vi "Sweeping Turn.vi"(6 "upper angle limit":dbl, 8 "error in":errorcluster) -> (0 "error out":errorcluster)   [LabVIEW 2017]
uses:
  Documents/LabVIEW Data/Retro 2018/Robot Global Data.vi
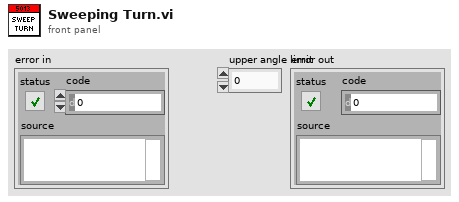
[diagram p1: front panel]
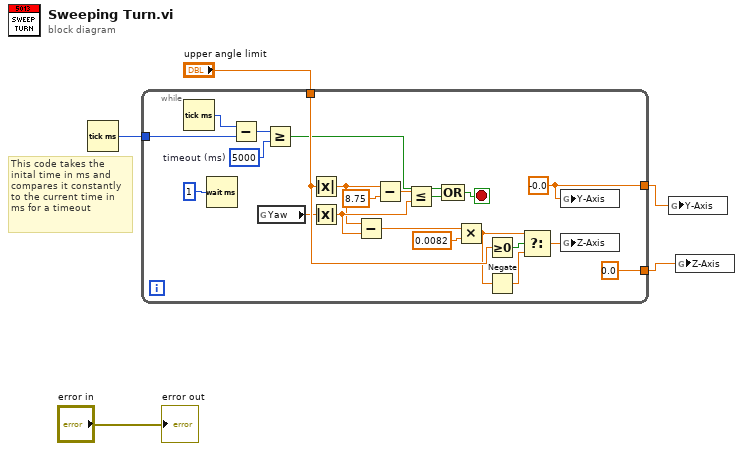
[diagram p0: block diagram]
diagram:
  # "This code takes the\ninital time in ms and\ncompares it constantly\nto the current time in\nms for a timeout"
  n1 = Tick Count (ms)() -> (millisecond timer value=w1:u32)
  n2 = while {
    tunnel: "upper angle limit" -> [w24]
    tunnel: [0.0 ("setpoint")] -> w3
    tunnel: [w17] -> w2
    tunnel: w1 -> [w10]
    stop <- w8 stop-if-true
    w6 = u32 5000  # timeout (ms)
    w17 = -0.0 ("Y-Axis")
    n3 = Tick Count (ms)() -> (millisecond timer value=w11:u32)
    n4 = Wait (ms)(milliseconds to wait=u32 1) -> ()  [unwired: 1 out]
    n5 = Subtract(x=w11, y=w10) -> (x-y=w9:u32)
    n6 = global read "Robot Global Data.vi" "Yaw"() -> (w18:dbl)
    n7 = Greater Or Equal?(x=w9, y=w6) -> (x >= y?=w7:bool)
    n8 = Absolute Value(x=w24) -> (abs(x)=w15:dbl)
    n9 = Absolute Value(x=w18) -> (abs(x)=w16:dbl)
    n10 = Subtract(x=w15, y=w16) -> (x-y=w14:dbl)
    n11 = Subtract(x=w15, y=8.75 ("x")) -> (x-y=w20:dbl)
    n12 = Less Or Equal?(x=w20, y=w16) -> (x <= y?=w25:bool)
    n13 = Compound Arithmetic op=OR(w7, w25) -> (w8:bool)
    n14 = Multiply(x=w14, y=0.0082 ("Y-Axis")) -> (x*y=w12:dbl)
    n15 = Greater Or Equal To 0?(x=w24) -> (x >= 0?=w23:bool)
    n16 = Negate(x=w12) -> (-x=w22:dbl)
    n17 = Select(t=w12, s=w23, f=w22) -> (s? t:f=w21:dbl)
    n18 = global write "Robot Global Data.vi" "Y-Axis"(w17) -> ()
    n19 = global write "Robot Global Data.vi" "Z-Axis"(w21) -> ()
  }
  n20 = global write "Robot Global Data.vi" "Y-Axis"(w2) -> ()
  n21 = global write "Robot Global Data.vi" "Z-Axis"(w3) -> ()
  "error out" <- "error in"
